vi "Mixer.Close.vi"() -> (0 "success":bool)   [LabVIEW 2020]
uses:
  <vilib>/Utility/sysdir.llb/System Directory Type.ctl
  <vilib>/Utility/config.llb/Write Key (I32).vi
  <vilib>/Utility/config.llb/NI_LVConfig.lvlib
panel:
  out "error out":errorcluster
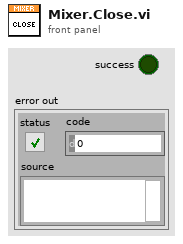
[diagram p1: front panel]
types:
  T1 = enum32{"Bad", "Idle", "Run top level", "Running"}
  T2 = typedef "System Directory Type.ctl" = i32
  T3 = typedef "LVRectTypeDef.ctl" = cluster{"Left":i16, "Top":i16, "Right":i16, "Bottom":i16}
  T4 = typedef "NI_LVConfig.lvlib/Config Data RefNum.ctl" = refnum<k1>
  T5 = enum32{"Invalid", "Standard", "Closed", "Hidden", "Minimized", "Maximized"}
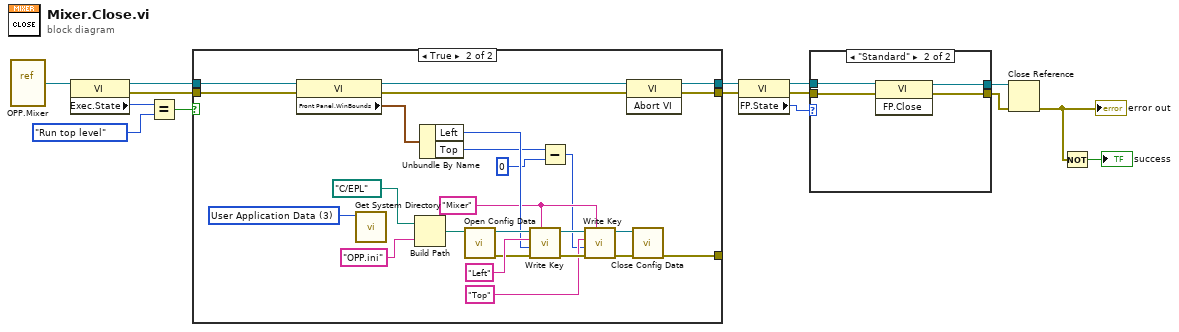
[diagram p0: block diagram]
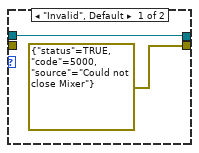
[diagram p2: hidden frame]
diagram:
  n1 = vi-ref "OPP.Mixer.vi"() -> (w12:refnum<vi>)
  n2 = property class="VI"(reference=w12) -> (reference out=w15:refnum<vi>, error out=w14:errorcluster, "Exec.State"=w11:T1)  [unwired: 1 in]
  n3 = Equal?(x=w11, y=T1."Run top level" ("Execution:State")) -> (x = y?=w10:bool)
  n4 = case shown="True" w10 {
    tunnel: w15 -> [w17 w40]
    tunnel: w14 -> [w16 w39]
    tunnel: [w17 w42] -> w7
    tunnel: [w16 w41] -> w6
    tunnel: [_ w21] -> _
    frame False {
    }
    frame True {
      w26 = "Mixer" ("section")
      w35 = T2 3 items=["User Home"=0, "User Desktop"=1, "User Documents"=2, "User Application Data"=3, "User Preferences"=4, "User Temporary"=5, "Public Documents"=6, "Public Application Data"=7, "Public Preferences"=8, "Public Cache"=13, "System Core Libraries"=9, "System Installed Libraries"=10, "Application Files"=11, "Boot Volume Root"=12] ("system directory type")
      n5 = property class="VI"(reference=w40, error in=w39) -> (reference out=w38:refnum<vi>, error out=w37:errorcluster, "Front Panel.WinBounds"=w36:T3)
      n6 = call <vilib>:"Get System Directory.vi"("system directory type"=w35) -> ()  [unwired: 10 in, 1 out]
      n7 = Build Path(base path=path "C:/EPL", name or relative path="OPP.ini") -> (appended path=w33:path)
      n8 = Unbundle By Name(w36) -> ("Left"=w30:i16, "Top"=w25:i16)
      n9 = call <vilib>:"Open Config Data.vi"("configuration file path"=w33) -> ("error out"=w28:errorcluster, "refnum"=w32:T4)  [unwired: 8 in, 1 out]
      n10 = call-poly <vilib>:"Write Key.vi"("section"=w26, "error in (no error)"=w28, "value"=w30, "key"="Left", "refnum"=w32) -> ("error out"=w27:errorcluster, "refnum out"=w29:T4)  [unwired: 4 in, 1 out]
      n11 = Subtract(x=w25, y=i16 0) -> (x-y=w20:i16)
      n12 = call-poly <vilib>:"Write Key.vi"("section"=w26, "error in (no error)"=w27, "value"=w20, "key"="Top", "refnum"=w29) -> ("error out"=w23:errorcluster, "refnum out"=w22:T4)  [unwired: 4 in, 1 out]
      n13 = invoke class="VI" method="Abort VI"(reference=w38, error in=w37) -> (reference out=w42:refnum<vi>, error out=w41:errorcluster)  [unwired: 1 in, 1 out]
      n14 = call <vilib>:"Close Config Data.vi"("error in (no error)"=w23, "refnum"=w22) -> ("error out"=w21:errorcluster)  [unwired: 8 in, 1 out]
    }
  }
  n15 = property class="VI"(reference=w7, error in=w6) -> (reference out=w5:refnum<vi>, error out=w1:errorcluster, "FP.State"=w4:T5)
  n16 = case shown="\"Standard\"" w4 {
    tunnel: [w43 w48] -> w3
    tunnel: [errorcluster {"status"=TRUE, "code"=5000, "source"="Could not close Mixer"} ("error out") w47] -> w2
    tunnel: w5 -> [w43 w46]
    tunnel: w1 -> [_ w45]
    frame "Invalid", Default {
    }
    frame "Standard" {
      n17 = invoke class="VI" method="FP.Close"(reference=w46, error in=w45) -> (reference out=w48:refnum<vi>, error out=w47:errorcluster)  [unwired: 1 in, 1 out]
    }
  }
  n18 = Close Reference(reference=w3, error in (no error)=w2) -> (error out=w8:errorcluster)
  "error out" <- w8
  n19 = Not(x=w8) -> (.not. x?=→"success":bool)
